vi "Set pressed button green.vi"(6 "Init":bool, 8 "error in (no error)":errorcluster, 10 "Controll collection":T1, 11 "Selected control":refnum<vi>) -> (0 "error out":errorcluster)   [LabVIEW 2011]
doc: "Resets all bundled command buttons to grey except the pressed button which is set to green."
uses:
  Controll refrence groups.ctl
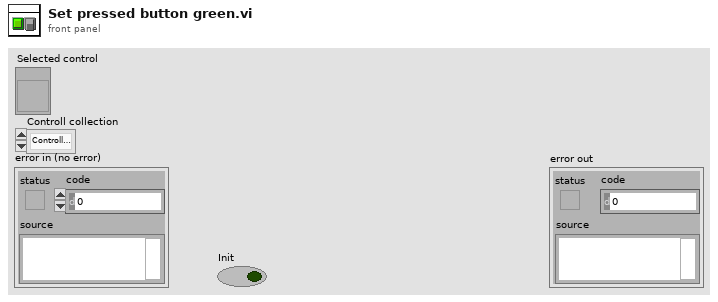
[diagram p1: front panel]
types:
  T1 = typedef "Controll refrence groups.ctl" = enum16{"Controller. gen", "Controller . High G", "Stroker", "PCP Online", "PCP Local", "PCP HV On", "Driller", "Stroker Cmd Buttons", "Stroker Anchor Cmd Buttons", "Controller Relay Buttons", "PCP Start Telemetry", "PCP Start Motor", "Tractor", "Modem Status"}
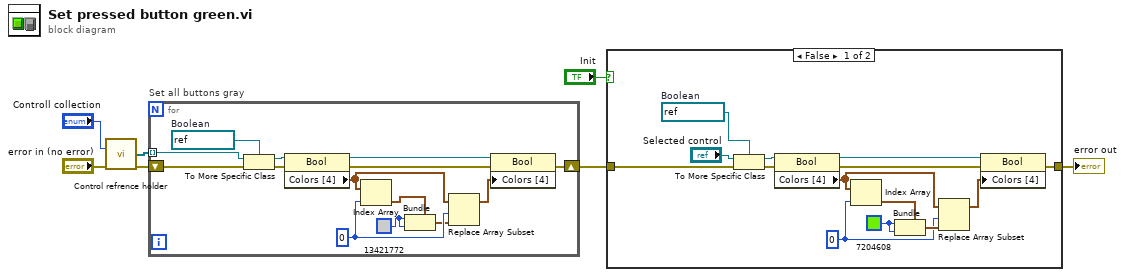
[diagram p0: block diagram]
diagram:
  n1 = call "Control refrence holder.vi"("Controll collection"="Controll collection", "error in (no error)"="error in (no error)") -> ("Controlls out"=w6:refnum<vi>[], "error out"=w5:errorcluster)  [unwired: 12 in]
  n2 = for "Set all buttons gray" {
    tunnel: w6 -> [w16] mode=indexing
    shift-right: [w9] -> w4
    shift-left: w5 -> [w12]
    w14 = refnum<vi> refnum  # Boolean
    w20 = 0 ("index")
    w8 = u32 13421772
    n3 = To More Specific Class(target class=w14, reference=w16, error in=w12) -> (specific class reference=w15:refnum<vi>, error out=w11:errorcluster)
    n4 = property on="Property Node" class="Bool"(reference=w15, error in=w11) -> (reference out=w13:refnum<vi>, error out=w10:errorcluster, "Colors [4]"=w18:cluster{u32, u32}[])
    n5 = Index Array(array=w18, index=w20) -> (element=w17:cluster{u32, u32})
    n6 = Bundle(cluster=w17, w8, w8) -> (w19:cluster{u32, u32})
    n7 = Replace Array Subset(array=w18, new element=w19, index=w20) -> (w21:cluster{u32, u32}[])
    n8 = property on="Property Node" class="Bool"(reference=w13, error in=w10, "Colors [4]"=w21) -> (error out=w9:errorcluster)  [unwired: 1 out]
  }
  n9 = case shown="False" "Init" {
    tunnel: w4 -> [w25 w36]
    tunnel: [w22 w36] -> w1
    frame False {
      w32 = refnum<vi> refnum  # Boolean
      w27 = 0 ("index")
      w23 = u32 7204608
      n10 = To More Specific Class(target class=w32, reference="Selected control", error in=w25) -> (specific class reference=w31:refnum<vi>, error out=w34:errorcluster)
      n11 = property on="Property Node" class="Bool"(reference=w31, error in=w34) -> (reference out=w33:refnum<vi>, error out=w35:errorcluster, "Colors [4]"=w29:cluster{u32, u32}[])
      n12 = Index Array(array=w29, index=w27) -> (element=w30:cluster{u32, u32})
      n13 = Bundle(cluster=w30, w23, w23) -> (w28:cluster{u32, u32})
      n14 = Replace Array Subset(array=w29, new element=w28, index=w27) -> (w26:cluster{u32, u32}[])
      n15 = property on="Property Node" class="Bool"(reference=w33, error in=w35, "Colors [4]"=w26) -> (error out=w22:errorcluster)  [unwired: 1 out]
    }
    frame True {
      # "Init case will make sure that all controls are gray"
    }
  }
  "error out" <- w1
